vi "configure_rx_transfer_group.vi"(11 "RX Transfer Group":T12={"Timing"={"priority"=100, "decimation"=1, "offset"=0}, "RX Connections"=[]}) -> (3 "Transfer Group Configuration":T1={"core"={"name"="Group", "direction"=enum."Tx", "cycle timing"={"priority"=100, "decimation"=1, "offset"=0}, "timeout behavior"=enum."Increment Late Count", "enable conversion"=FALSE}, "component settings"=[], "transfers"=[]} {"transfers"."channels"."core"."string offset" format="%d bytes"})   [LabVIEW 2020]
uses:
  controls/rx_configuration_data.ctl
  <vilib>/addons/VeriStand Custom Device Scripting APIs/Data Sharing Framework/DSF Core.lvlibp/Typedefs/DSF Timing Info.ctl
  <vilib>/addons/VeriStand Custom Device Scripting APIs/Data Sharing Framework/DSF Core.lvlibp/Typedefs/DSF Settings Info.ctl
  <vilib>/addons/VeriStand Custom Device Scripting APIs/Data Sharing Framework/DSF Core.lvlibp
  <vilib>/addons/VeriStand Custom Device Scripting APIs/Data Sharing Framework/DSF Core.lvlibp/Typedefs/DSF Data Type.ctl
  <vilib>/addons/VeriStand Custom Device Scripting APIs/Data Sharing Framework/DSF Core.lvlibp/Typedefs/Core Channel Configuration.ctl
  <vilib>/addons/VeriStand Custom Device Scripting APIs/Data Sharing Framework/DSF Core.lvlibp/Classes/Configuration/Core/Channel/Channel Configuration.lvclass
  <vilib>/addons/VeriStand Custom Device Scripting APIs/Data Sharing Framework/DSF Core.lvlibp/Typedefs/DSF Engine Channel Configuration.ctl
  <vilib>/addons/VeriStand Custom Device Scripting APIs/Data Sharing Framework/DSF Core.lvlibp/Typedefs/Core Transfer Configuration.ctl
  <vilib>/addons/VeriStand Custom Device Scripting APIs/Data Sharing Framework/DSF Core.lvlibp/Classes/Configuration/Core/Transfer/Transfer Configuration.lvclass
  <vilib>/addons/VeriStand Custom Device Scripting APIs/Data Sharing Framework/DSF Core.lvlibp/Typedefs/DSF Engine Transfer Configuration.ctl
  <vilib>/addons/VeriStand Custom Device Scripting APIs/Data Sharing Framework/DSF Core.lvlibp/Typedefs/DSF Timeout Behavior.ctl
  <vilib>/addons/VeriStand Custom Device Scripting APIs/Data Sharing Framework/DSF Core.lvlibp/Typedefs/DSF Direction.ctl
  <vilib>/addons/VeriStand Custom Device Scripting APIs/Data Sharing Framework/DSF Core.lvlibp/Typedefs/Core Group Configuration.ctl
  <vilib>/addons/VeriStand Custom Device Scripting APIs/Data Sharing Framework/DSF Core.lvlibp/Classes/Configuration/Core/Group/Group Configuration.lvclass
  <vilib>/addons/VeriStand Custom Device Scripting APIs/Data Sharing Framework/DSF Core.lvlibp/Typedefs/DSF Engine Transfer Group Configuration.ctl
  controls/rx_transfer_group_configuration_data.ctl
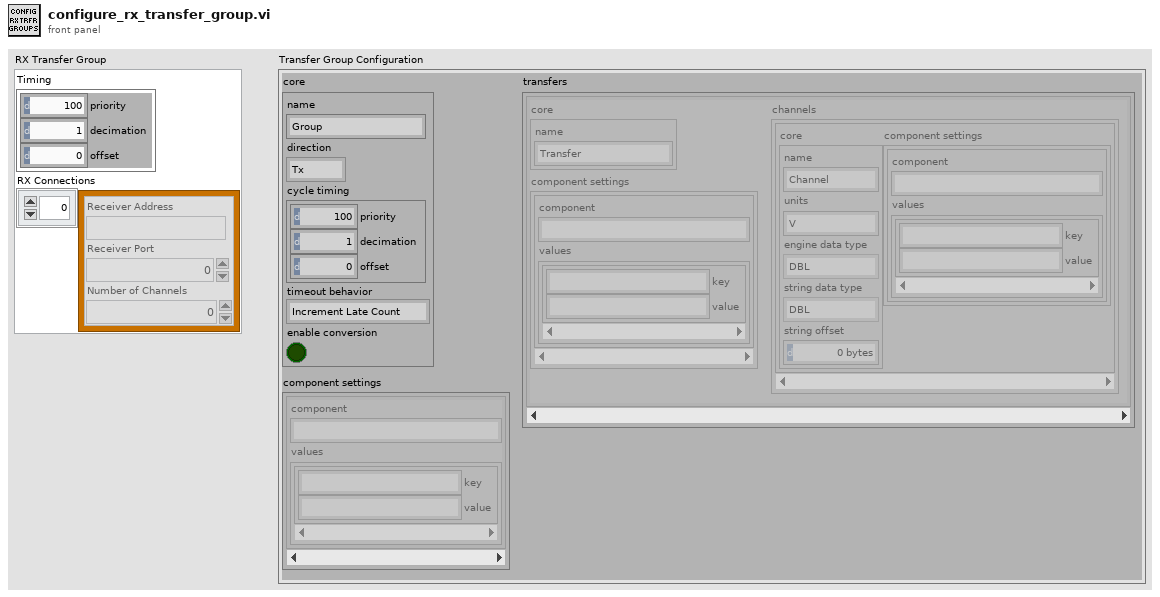
[diagram p1: front panel]
types:
  T1 = typedef "DSF Core.lvlibp/DSF Engine Transfer Group Configuration.ctl" = cluster{"core":T2, "component settings":T6[], "transfers":T7[]}
  T2 = typedef "DSF Core.lvlibp/Group Configuration.lvclass/Core Group Configuration.ctl" = cluster{"name":string, "direction":T3, "cycle timing":T4, "timeout behavior":T5, "enable conversion":bool}
  T3 = typedef "DSF Core.lvlibp/DSF Direction.ctl" = enum8{"Tx", "Rx"}
  T4 = typedef "DSF Core.lvlibp/DSF Timing Info.ctl" = cluster{"priority":u64, "decimation":u64, "offset":u64}
  T5 = typedef "DSF Core.lvlibp/DSF Timeout Behavior.ctl" = enum8{"Increment Late Count", "Throw Error"}
  T6 = typedef "DSF Core.lvlibp/DSF Settings Info.ctl" = cluster{"component":string, "values":cluster{"key":string, "value":string}[]}
  T7 = typedef "DSF Core.lvlibp/DSF Engine Transfer Configuration.ctl" = cluster{"core":T8, "component settings":T6[], "channels":T9[]}
  T8 = typedef "DSF Core.lvlibp/Transfer Configuration.lvclass/Core Transfer Configuration.ctl" = cluster{"name":string}
  T9 = typedef "DSF Core.lvlibp/DSF Engine Channel Configuration.ctl" = cluster{"core":T10, "component settings":T6[]}
  T10 = typedef "DSF Core.lvlibp/Channel Configuration.lvclass/Core Channel Configuration.ctl" = cluster{"name":string, "units":string, "engine data type":T11, "string data type":T11, "string offset":u64}
  T11 = typedef "DSF Core.lvlibp/DSF Data Type.ctl" = enum8{"Bool", "SGL", "DBL", "I8", "I16", "I32", "I64", "U8", "U16", "U32", "U64"}
  T12 = typedef "rx_transfer_group_configuration_data.ctl" = cluster{"Timing":T4, "RX Connections":T13[]}
  T13 = typedef "rx_configuration_data.ctl" = cluster{"Receiver Address":string, "Receiver Port":u16, "Number of Channels":u16}
  T14 = cluster{"component":string, "values":cluster{"key":string, "value":string}[]}[]
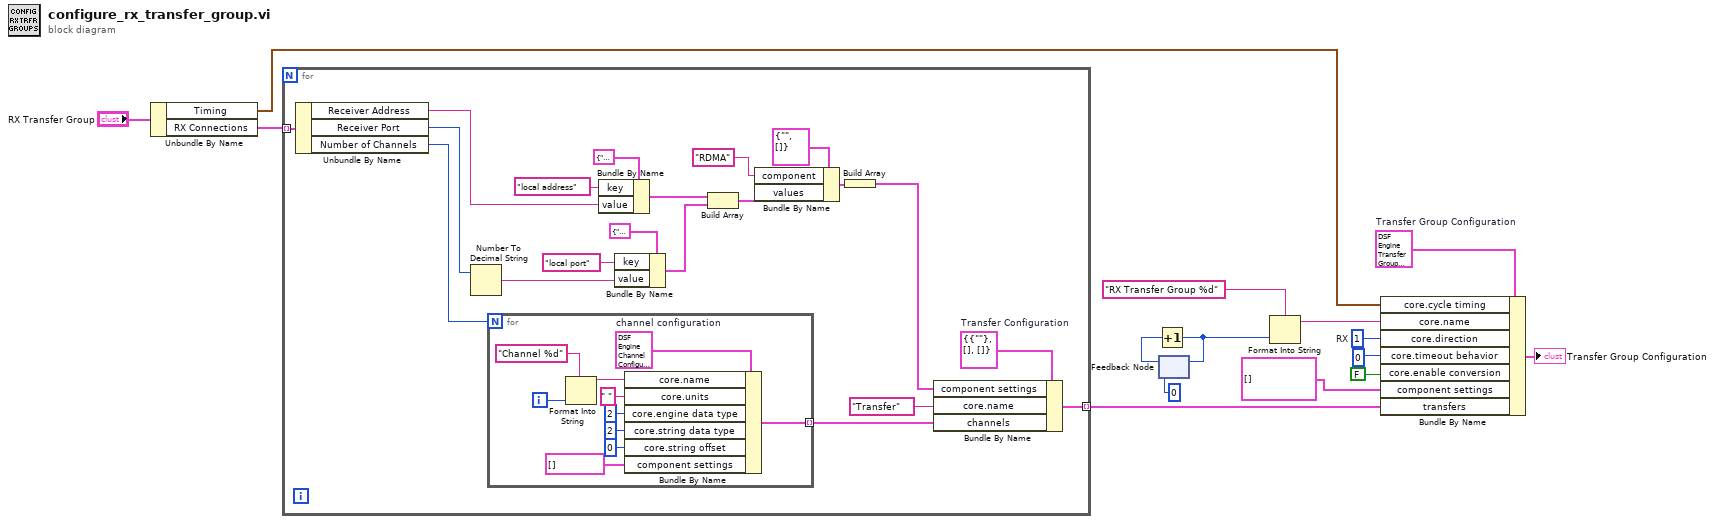
[diagram p0: block diagram]
diagram:
  w13 = T1 {"core"={"name"="", "direction"=enum."Tx", "cycle timing"={"priority"=0, "decimation"=0, "offset"=0}, "timeout behavior"=enum."Increment Late Count", "enable conversion"=FALSE}, "component settings"=[], "transfers"=[]}  # Transfer Group Configuration
  w9 = u32 1  # RX
  n1 = Unbundle By Name("RX Transfer Group") -> ("Timing"=w2:T4, "RX Connections"=w14:T13[])
  n2 = for {
    tunnel: w14 -> [w35] mode=indexing
    tunnel: [w16] -> w6 mode=indexing
    w18 = T7 {"core"={"name"=""}, "component settings"=[], "channels"=[]}  # Transfer Configuration
    n3 = Unbundle By Name(w35) -> ("Receiver Address"=w30:string, "Receiver Port"=w29:u16, "Number of Channels"=w22:u16)
    n4 = Number To Decimal String(number=w29) -> (decimal integer string=w31:string)  [unwired: 1 in]
    n5 = for {
      N: w22 -> [_]
      tunnel: [w45] -> w21 mode=indexing
      i -> [w43]
      w36 = T9 {"core"={"name"="Channel", "units"="V", "engine data type"=enum."DBL", "string data type"=enum."DBL", "string offset"=0}, "component settings"=[]}  # channel configuration
      n6 = Format Into String(format string="Channel %d", w43) -> (resulting string=w42:string)  [unwired: 2 in, 1 out]
      n7 = Bundle By Name(cluster=w36, "core.name"=w42, "core.units"=" ", "core.engine data type"=u8 2, "core.string data type"=u8 2, "core.string offset"=u8 0, "component settings"=T14 []) -> (w45:T9)
    }
    n8 = Bundle By Name(cluster=cluster{"key":string, "value":string} {"key"="", "value"=""} ("value"), "key"="local address", "value"=w30) -> (w26:cluster{"key":string, "value":string})
    n9 = Bundle By Name(cluster=cluster{"key":string, "value":string} {"key"="", "value"=""} ("value"), "key"="local port", "value"=w31) -> (w25:cluster{"key":string, "value":string})
    n10 = Build Array(w26, w25) -> (w24:cluster{"key":string, "value":string}[])
    n11 = Bundle By Name(cluster=T6 {"component"="", "values"=[]} ("component settings"), "component"="RDMA", "values"=w24) -> (w23:T6)
    n12 = Build Array(w23) -> (w20:T6[])
    n13 = Bundle By Name(cluster=w18, "component settings"=w20, "core.name"="Transfer" ("format string"), "channels"=w21) -> (w16:T7)
  }
  n14 = feedback #1(0) -> (w4:i32)
  n15 = Increment(x=w4) -> (x+1=w3:i32)
  n16 = feedback-in #1(w3) -> ()
  n17 = Format Into String(format string="RX Transfer Group %d", w3) -> (resulting string=w8:string)  [unwired: 2 in, 1 out]
  n18 = Bundle By Name(cluster=w13, "core.cycle timing"=w2, "core.name"=w8, "core.direction"=w9, "core.timeout behavior"=u32 0, "core.enable conversion"=FALSE, "component settings"=T6[] [], "transfers"=w6) -> (→"Transfer Group Configuration":T1)
